vi "CRYDB Insert Into ValueTable.vi"(0 "connection reference":T2, 1 "Curve_ID":u32, 2 "Value":dbl[](array[numeric]), 3 "error in":errorcluster) -> (7 "connection reference out":T2, 10 "error out":errorcluster)   [LabVIEW 2013]
uses:
  <vilib>/addons/database/Connection.llb/Conn ObjectReference.ctl
  <vilib>/addons/database/Auxilliary.llb/DB Tools Column Info.ctl
  <vilib>/addons/database/Auxilliary.llb/DB Tools DataTypes.ctl
  <vilib>/addons/database/NI_Database_API.lvlib
panel:
  in  "Table":T1
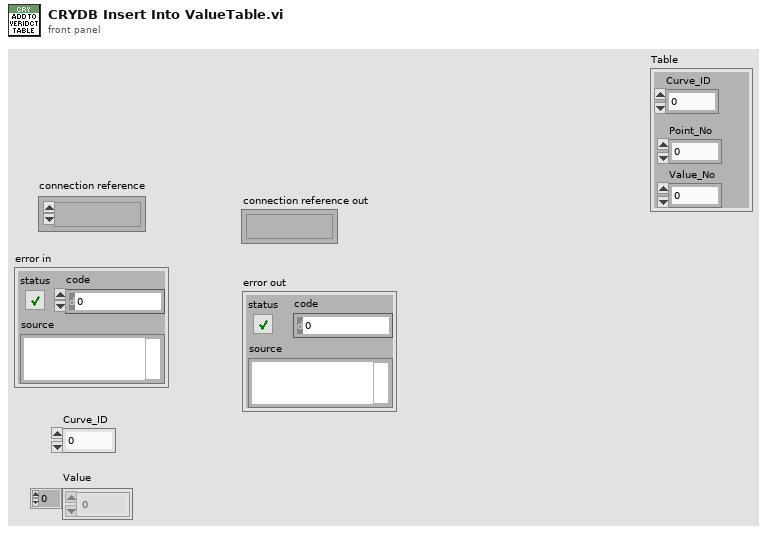
[diagram p1: front panel]
types:
  T1 = cluster{"Curve_ID":u32, "Point_No":u32, "Value_No":dbl}
  T2 = typedef "NI_Database_API.lvlib/Conn ObjectReference.ctl" = refnum<k1>
  T3 = typedef "NI_Database_API.lvlib/DB Tools Column Info.ctl" = cluster{"column name":string, "data type":T4, "size":i32, "allow null?":bool}
  T4 = typedef "NI_Database_API.lvlib/DB Tools DataTypes.ctl" = enum16{"String", "Long (I32)", "Single (SGL)", "Double (DBL)", "Date/Time", "Binary"}
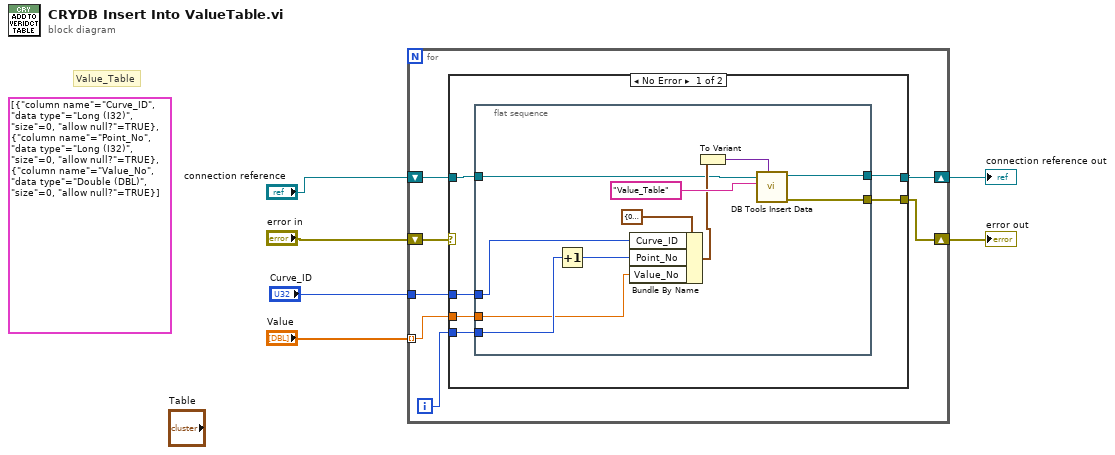
[diagram p0: block diagram]
diagram:
  (unwired) T3[] [{"column name"="Curve_ID", "data type"=enum."Long (I32)", "size"=0, "allow null?"=TRUE}, {"column name"="Point_No", "data type"=enum."Long (I32)", "size"=0, "allow null?"=TRUE}, {"column name"="Value_No", "data type"=enum."Double (DBL)", "size"=0, "allow null?"=TRUE}] ("column information")
  # "Value_Table"
  n1 = for {
    shift-right: [w10] -> w3
    shift-left: "connection reference" -> [w12]
    shift-right: [w11] -> w4
    shift-left: "error in" -> [w13]
    tunnel: "Value" -> [w9] mode=indexing
    tunnel: "Curve_ID" -> [w8]
    i -> [w7]
    n2 = case shown="No Error" w13 {
      selector: w13 -> [_ w31]
      tunnel: w12 -> [w17 w32]
      tunnel: [w19 w32] -> w10
      tunnel: [w18 w31] -> w11
      tunnel: w9 -> [w16 _]
      tunnel: w8 -> [w15 _]
      tunnel: w7 -> [w14 _]
      frame No Error {
        n3 = flat-sequence {
          tunnel: [w30] -> w19
          tunnel: [w29] -> w18
          tunnel: w17 -> [w25]
          tunnel: w16 -> [w21]
          tunnel: w15 -> [w23]
          tunnel: w14 -> [w22]
          frame #0 {
            n4 = Increment(x=w22) -> (x+1=w20:i32)
            n5 = Bundle By Name(cluster=T1 {"Curve_ID"=0, "Point_No"=0, "Value_No"=0.0} ("Table"), "Curve_ID"=w23, "Point_No"=w20, "Value_No"=w21) -> (w26:T1)
            n6 = To Variant(anything=w26) -> (Variant=w27:variant)
            n7 = call <vilib>:"DB Tools Insert Data.vi"("data"=w27, "table"="Value_Table", "connection reference"=w25) -> ("error out"=w29:errorcluster, "connection reference out"=w30:T2)  [unwired: 7 in]
          }
        }
      }
      frame Error {
      }
    }
  }
  "connection reference out" <- w3
  "error out" <- w4
